vi "Join Strings.vi"(0 "string array":string[](array[string]), 5 "separator":string=" ") -> (4 "string out":string)   [LabVIEW 2015, in "LV String Utils v1.lvlib"]
doc: "Inspired by 'join' method of string class in Python."
uses:
  LV String Utils v1.lvlib
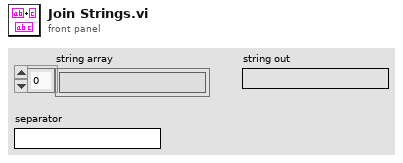
[diagram p1: front panel]
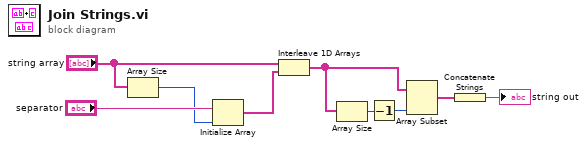
[diagram p0: block diagram]
diagram:
  n1 = Array Size(array="string array") -> (size(s)=w5:i32)
  n2 = Initialize Array("separator", w5) -> (w7:string[])
  n3 = Interleave 1D Arrays("string array", w7) -> (w4:string[])
  n4 = Array Size(array=w4) -> (size(s)=w3:i32)
  n5 = Decrement(x=w3) -> (x-1=w2:i32)
  n6 = Array Subset(array=w4, length=w2) -> (w1:string[])  [unwired: 1 in]
  n7 = Concatenate Strings(w1) -> (→"string out":string)
